vi "Day.vi"() -> ()   [LabVIEW 2021]
uses:
  <vilib>/addons/_JKI Toolkits/Caraya/classes/Assert/Assert Equal Value_Variant.vi
  <vilib>/addons/_JKI Toolkits/Caraya/classes/Assert/Assert.lvclass
  <vilib>/addons/_JKI Toolkits/Caraya/classes/Test/Test.lvclass
panel:
  out "Solution Part 2":i64
  out "Solution Part 1":i64
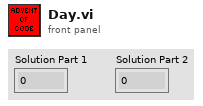
[diagram p1: front panel]
types:
  T1 = cluster{"Result Part1":dbl, "Result Part2":dbl, "Input":string}
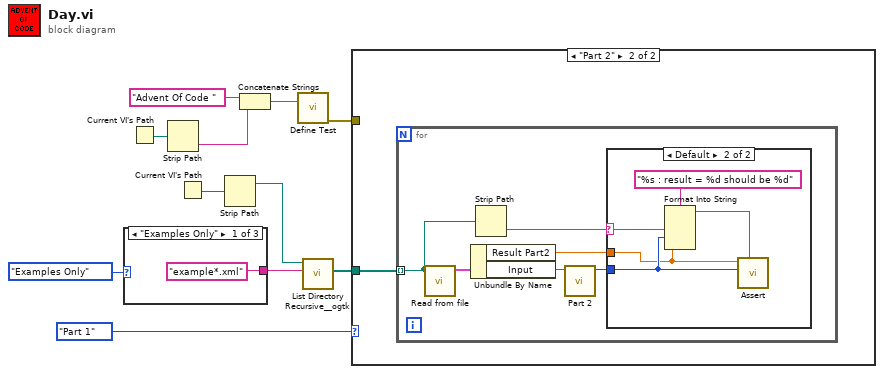
[diagram p0: block diagram]
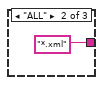
[diagram p2: hidden frame]
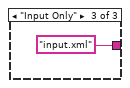
[diagram p3: hidden frame]
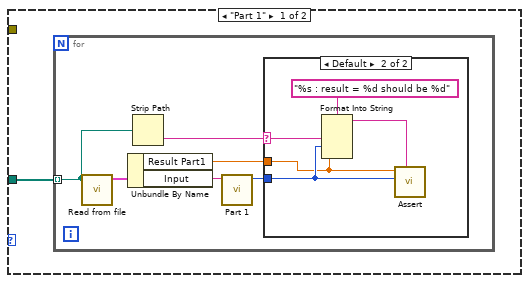
[diagram p4: hidden frame]
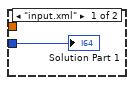
[diagram p5: hidden frame]
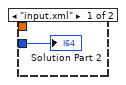
[diagram p6: hidden frame]
diagram:
  n1 = case shown="\"Examples Only\"" enum16{"Examples Only", "ALL", "Input Only"}."Examples Only" ("Part 2") {
    tunnel: ["example*.xml" ("pattern") "*.xml" ("pattern") "input.xml" ("pattern")] -> w2
    frame "Examples Only" {
    }
    frame "ALL" {
    }
    frame "Input Only" {
    }
  }
  n2 = Current VI's Path() -> (path=w5:path)
  n3 = Strip Path(path=w5) -> (name=w3:string)  [unwired: 1 out]
  n4 = Current VI's Path() -> (path=w11:path)
  n5 = Strip Path(path=w11) -> (stripped path=w10:path)  [unwired: 1 out]
  n6 = Concatenate Strings("Advent Of Code " ("Label (VI Title)"), w3) -> (w4:string)
  n7 = call <vilib>:"Define Test.vi"("Label (VI Title)"=w4) -> ("error out"=w7:errorcluster)  [unwired: 10 in]
  n8 = call <userlib>:"List Directory Recursive__ogtk.vi"("pattern"=w2, "Path"=w10) -> ("file paths"=w8:path[])  [unwired: 6 in, 3 out]
  n9 = case shown="\"Part 2\"" enum16{"Part 1", "Part 2"}."Part 1" ("Part") {
    tunnel: w8 -> [w15 w28]
    tunnel: w7 -> [_ _]
    frame "Part 1" {
      n10 = for {
        tunnel: w15 -> [w18] mode=indexing
        n11 = call "Read from file.vi"("File Path"=w18) -> ("Data"=w20:T1)  [unwired: 10 in]
        n12 = Unbundle By Name(w20) -> ("Result Part1"=w19:dbl, "Input"=w21:string)
        n13 = Strip Path(path=w18) -> (name=w17:string)  [unwired: 1 out]
        n14 = call "Part 1.vi"("Input"=w21) -> ("Output"=w16:i64)  [unwired: 10 in]
        n15 = case shown="Default" w17 {
          selector: w17 -> [_ w27]
          tunnel: w19 -> [_ w23]
          tunnel: w16 -> [w22 w24]
          frame "input.xml" {
            "Solution Part 1" <- w22
          }
          frame Default {
            n16 = Format Into String(format string="%s : result = %d should be %d", w27, w24, w23) -> (resulting string=w26:string)  [unwired: 2 in, 1 out]
            n17 = call-poly <vilib>:"Assert.vi"("Label"=w26, "Y"=w24, "X"=w23) -> ()  [unwired: 8 in, 1 out]
          }
        }
      }
    }
    frame "Part 2" {
      n18 = for {
        tunnel: w28 -> [w31] mode=indexing
        n19 = call "Read from file.vi"("File Path"=w31) -> ("Data"=w33:T1)  [unwired: 10 in]
        n20 = Unbundle By Name(w33) -> ("Result Part2"=w32:dbl, "Input"=w34:string)
        n21 = Strip Path(path=w31) -> (name=w30:string)  [unwired: 1 out]
        n22 = call "Part 2.vi"("Input"=w34) -> ("Output"=w29:i64)  [unwired: 10 in]
        n23 = case shown="Default" w30 {
          selector: w30 -> [_ w40]
          tunnel: w32 -> [_ w36]
          tunnel: w29 -> [w35 w37]
          frame "input.xml" {
            "Solution Part 2" <- w35
          }
          frame Default {
            n24 = Format Into String(format string="%s : result = %d should be %d", w40, w37, w36) -> (resulting string=w39:string)  [unwired: 2 in, 1 out]
            n25 = call-poly <vilib>:"Assert.vi"("Label"=w39, "Y"=w37, "X"=w36) -> ()  [unwired: 8 in, 1 out]
          }
        }
      }
    }
  }
